vi "Trigger count.vi"(7 "reset":bool, 10 "total to read":i32, 11 "# read":i32) -> (3 "done?":bool)   [LabVIEW 2023]
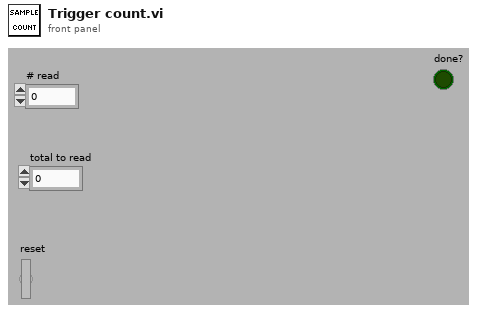
[diagram p1: front panel]
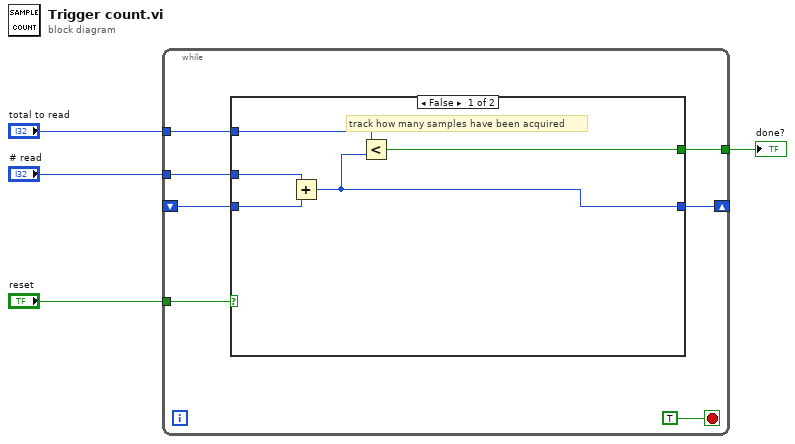
[diagram p0: block diagram]
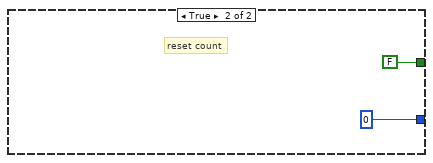
[diagram p2: hidden frame]
diagram:
  n1 = while {
    shift-right: [w9] -> _
    shift-left: _ -> [w7]
    tunnel: "reset" -> [w10]
    tunnel: "# read" -> [w8]
    tunnel: "total to read" -> [w6]
    tunnel: [w5] -> w1
    stop <- TRUE stop-if-true
    n2 = case shown="False" w10 {
      tunnel: [w12 0] -> w9
      tunnel: w8 -> [w16 _]
      tunnel: w7 -> [w15 _]
      tunnel: w6 -> [w14 _]
      tunnel: [w13 FALSE] -> w5
      frame False {
        # "track how many samples have been acquired"
        n3 = Add(x=w16, y=w15) -> (x+y=w12:i32)
        n4 = Less?(x=w14, y=w12) -> (x < y?=w13:bool)
      }
      frame True {
        # "reset count"
      }
    }
  }
  "done?" <- w1
